vi "FailureDescription.vi"(8 "error in (no error)":errorcluster, 10 "Actual":variant, 11 "Binary Operator in":refnum<class "Binary Operator.lvclass">) -> (0 "error out":errorcluster, 2 "Failure Description":string, 3 "Binary Operator out":refnum<class "Binary Operator.lvclass">)   [LabVIEW 2017, in "Transparent Assertions.lvlib" / "Binary Operator.lvclass"]
doc: "Return the second part of the scentence \"Failed asserting that ...\""
uses:
  Binary Operator.lvclass
  Binary Operator.lvclass/Binary Operator.ctl
  Constraint/Constraint.lvclass
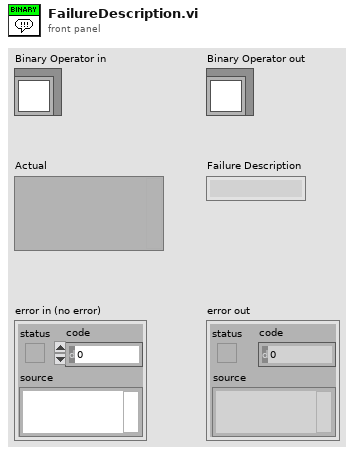
[diagram p1: front panel]
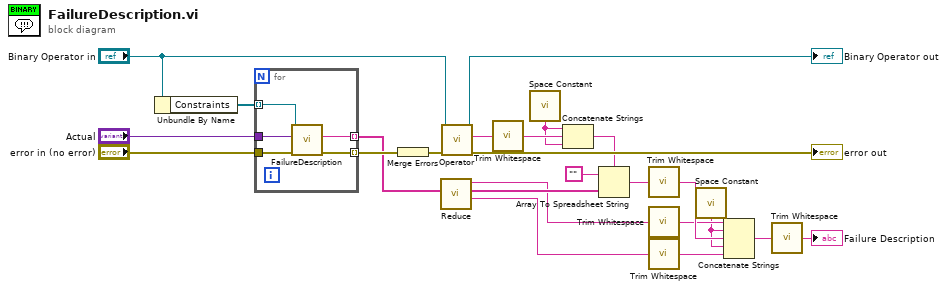
[diagram p0: block diagram]
diagram:
  n1 = Unbundle By Name("Binary Operator in") -> ("Constraints"=w22:refnum<class "Constraint.lvclass">[])
  n2 = for {
    tunnel: w22 -> [w27] mode=indexing
    tunnel: "error in (no error)" -> [w29]
    tunnel: [w28] -> w23 mode=indexing
    tunnel: [w26] -> w10 mode=indexing
    tunnel: "Actual" -> [w25]
    n3 = call-dynamic "FailureDescription.vi"("error in (no error)"=w29, "Actual"=w25, "Constraint in"=w27) -> ("error out"=w28:errorcluster, "Failure Description"=w26:string)  [unwired: 6 in, 1 out]
  }
  n4 = Merge Errors(w23) -> (w20:errorcluster)
  n5 = call "Reduce.vi"("Failure Descriptions"=w10) -> ("Suffix"=w3:string, "Failure Descriptions out"=w9:string[], "Prefix"=w7:string)  [unwired: 8 in]
  n6 = call-dynamic "Operator.vi"("error in (no error)"=w20, "Binary Operator in"="Binary Operator in") -> ("error out"=→"error out":errorcluster, "Operator"=w16:string, "Binary Operator out"=→"Binary Operator out":refnum<class "Binary Operator.lvclass">)  [unwired: 7 in]
  n7 = call <vilib>:"Trim Whitespace.vi"("string"=w16) -> ("trimmed string"=w14:string)  [unwired: 1 in]
  n8 = call <vilib>:"Space Constant.vi"() -> ("String"=w13:string)
  n9 = Concatenate Strings(w13, w14, w13) -> (w15:string)
  n10 = Array To Spreadsheet String(delimiter (Tab)=w15, array=w9, 3:"") -> (spreadsheet string=w12:string)
  n11 = call <vilib>:"Trim Whitespace.vi"("string"=w12) -> ("trimmed string"=w8:string)  [unwired: 1 in]
  n12 = call <vilib>:"Trim Whitespace.vi"("string"=w7) -> ("trimmed string"=w6:string)  [unwired: 1 in]
  n13 = call <vilib>:"Trim Whitespace.vi"("string"=w3) -> ("trimmed string"=w2:string)  [unwired: 1 in]
  n14 = call <vilib>:"Space Constant.vi"() -> ("String"=w4:string)
  n15 = Concatenate Strings(w6, w4, w8, w4, w2) -> (w5:string)
  n16 = call <vilib>:"Trim Whitespace.vi"("string"=w5) -> ("trimmed string"=→"Failure Description":string)  [unwired: 1 in]
